vi "Cross Correlation Compute.vi"(6 "Scale":dbl, 8 "normalization":enum32{"none", "unbiased", "biased"}(ring), 9 "algorithm":enum32{"direct", "frequency domain"}(ring), 10 "Waveform 2":waveform(dbl), 11 "Waveform 1":waveform(dbl)) -> (3 "Cross Correlation":cluster{dbl, "dt":dbl, dbl[]})   [LabVIEW 2017]
uses:
  <vilib>/Analysis/2dsp.llb/1D Cross Correlation (DBL).vi
  <vilib>/Analysis/NI_AALPro.lvlib
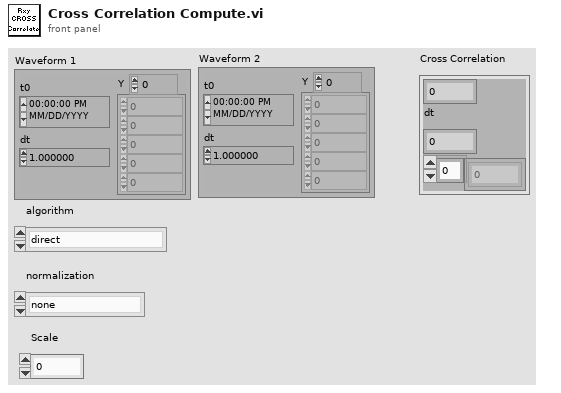
[diagram p1: front panel]
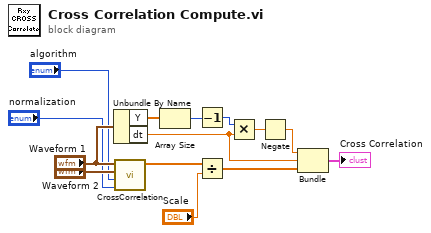
[diagram p0: block diagram]
diagram:
  n1 = Unbundle By Name("Waveform 1") -> ("Y"=w1:dbl[], "dt"=w6:dbl)
  n2 = call-poly <vilib>:"CrossCorrelation.vi"("normalization"="normalization", "algorithm"="algorithm", "Y"="Waveform 2", "X"="Waveform 1") -> ("Rxy"=w13:dbl[])  [unwired: 6 in, 1 out]
  n3 = Array Size(array=w1) -> (size(s)=w2:i32)
  n4 = Decrement(x=w2) -> (x-1=w3:i32)
  n5 = Divide(x=w13, y="Scale") -> (x/y=w14:dbl[])
  n6 = Multiply(x=w3, y=w6) -> (x*y=w4:dbl)
  n7 = Negate(x=w4) -> (-x=w5:dbl)
  n8 = Bundle(w5, "dt"=w6, w14) -> (→"Cross Correlation":cluster{dbl, "dt":dbl, dbl[]})  [unwired: 1 in]
